vi "Anti-backlashMovement.vi"(9 "Target position":dbl, 10 "Start position":dbl, 11 "Connection Cluster in":T1) -> (3 "Connection Cluster out":T1)   [LabVIEW 2013]
uses:
  Global.vi
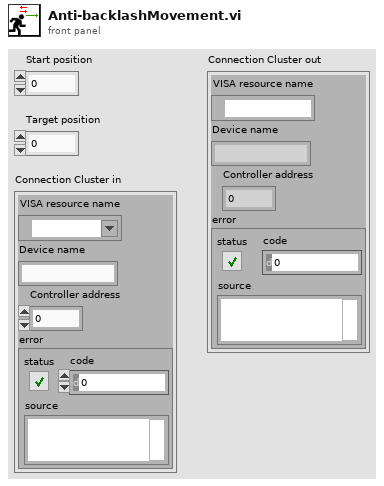
[diagram p1: front panel]
types:
  T1 = cluster{"VISA resource name":refnum<visa-resource-name>, "Device name":string, "Controller address":i32, "error":errorcluster}
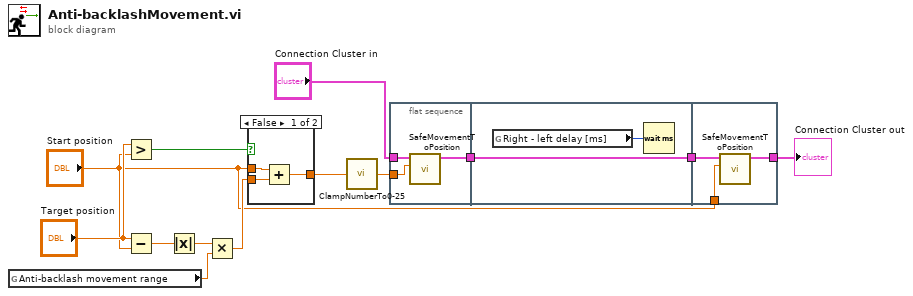
[diagram p0: block diagram]
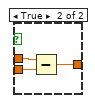
[diagram p2: hidden frame]
diagram:
  n1 = global read "Global.vi" "Anti-backlash movement range"() -> (w2:dbl)
  n2 = Greater?(x="Target position", y="Start position") -> (0:w10:bool)
  n3 = Subtract(x="Target position", y="Start position") -> (x-y=w11:dbl)
  n4 = Absolute Value(x=w11) -> (abs(x)=w12:dbl)
  n5 = Multiply(x=w12, y=w2) -> (x*y=w13:dbl)
  n6 = case shown="False" w10 {
    tunnel: "Start position" -> [w16 w18]
    tunnel: w13 -> [w15 w17]
    tunnel: [w14 w19] -> w4
    frame False {
      n7 = Add(x=w16, y=w15) -> (x+y=w14:dbl)
    }
    frame True {
      n8 = Subtract(x=w18, y=w17) -> (x-y=w19:dbl)
    }
  }
  n9 = call "ClampNumberTo0-25.vi"("Number"=w4) -> ("Clamped number"=w3:dbl)
  n10 = flat-sequence {
    tunnel: w3 -> [w22]
    tunnel: "Connection Cluster in" -> [w21]
    tunnel: [w20] -> w8
    tunnel: w8 -> [w24]
    tunnel: [w24] -> w7
    tunnel: w7 -> [w27]
    tunnel: "Start position" -> [w25]
    tunnel: [w26] -> w6
    frame #0 {
      n11 = call "SafeMovementToPosition.vi"("Target position"=w22, "Connection Cluster in"=w21) -> ("Connection Cluster out"=w20:T1)  [unwired: 9 in]
    }
    frame #1 {
      n12 = global read "Global.vi" "Right - left delay [ms]"() -> (w23:i32)
      n13 = Wait (ms)(milliseconds to wait=w23) -> ()  [unwired: 1 out]
    }
    frame #2 {
      n14 = call "SafeMovementToPosition.vi"("Target position"=w25, "Connection Cluster in"=w27) -> ("Connection Cluster out"=w26:T1)  [unwired: 9 in]
    }
  }
  "Connection Cluster out" <- w6
